vi "testset_Continuous Acquisition.vi"(8 "error in":errorcluster, 11 "camera handle in":u64) -> (0 "error out":errorcluster, 3 "camera handle out":u64, 4 "Running after Stop?":bool, 5 "Running after Start?":bool)   [LabVIEW 2019, in "PICam.lvlib"]
uses:
  PICam.lvlib
  types/PicamAcquisitionErrorsMask.ctl
panel:
  out "readout_rate":dbl
  out "errors":T1
  out "running":bool
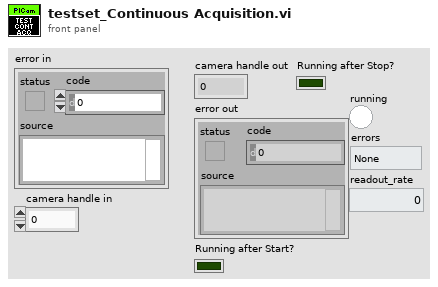
[diagram p1: front panel]
types:
  T1 = typedef "PicamAcquisitionErrorsMask.ctl" = enum8{"None", "DataLost", "ConnectionLost", "3", "DataNotArriving", "5", "6", "7", "ShutterOverheated", "9", "10", "11", "12", "13", "14", "15", "CameraFaulted"}
  T2 = typedef "PicamAcquisitionStatus.ctl" = cluster{"running":bool, "errors":T1, "readout_rate":dbl}
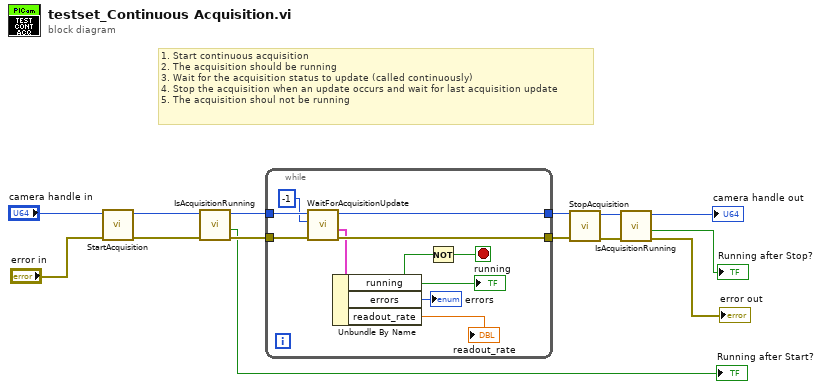
[diagram p0: block diagram]
diagram:
  # "1. Start continuous acquisition\n2. The acquisition should be running\n3. Wait for the acquisition status to update (called continuously)\n4. Stop the acquisition when an update occurs and wait for last acquisition update\n5. The acquisition shoul not be running"
  n1 = call "StartAcquisition.vi"("error in"="error in", "camera handle in"="camera handle in") -> ("error out"=w11:errorcluster, "camera handle out"=w14:u64)  [unwired: 8 in]
  n2 = call "IsAcquisitionRunning.vi"("error in"=w11, "camera handle in"=w14) -> ("error out"=w10:errorcluster, "IsAcquisitionRunning"=→"Running after Start?":bool, "camera handle out"=w13:u64)  [unwired: 7 in]
  n3 = while {
    tunnel: w10 -> [w22]
    tunnel: [w21] -> w9
    tunnel: w13 -> [w24]
    tunnel: [w23] -> w12
    stop <- w15 stop-if-true
    n4 = call "WaitForAcquisitionUpdate.vi"("error in (no error)"=w22, "piint (readout_time_out)"=i64 -1, "camera handle in"=w24) -> ("error out"=w21:errorcluster, "PicamAcquisitionStatus* status"=w19:T2, "camera handle out"=w23:u64)  [unwired: 5 in, 1 out]
    n5 = Unbundle By Name(w19) -> ("running"=w18:bool, "errors"=→"errors":T1, "readout_rate"=→"readout_rate":dbl)
    "running" <- w18
    n6 = Not(x=w18) -> (.not. x?=w15:bool)
  }
  n7 = call "StopAcquisition.vi"("error in"=w9, "camera handle in"=w12) -> ("error out"=w2:errorcluster, "camera handle out"=w1:u64)  [unwired: 8 in]
  n8 = call "IsAcquisitionRunning.vi"("error in"=w2, "camera handle in"=w1) -> ("error out"=→"error out":errorcluster, "IsAcquisitionRunning"=→"Running after Stop?":bool, "camera handle out"=→"camera handle out":u64)  [unwired: 7 in]
